vi "MISSION_ITEM Generic.vi"(11 "MISSION_ITEM":T1={"target_system"=0, "target_component"=0, "sequence"=0, "frame"=enum."GLOBAL RELATIVE ALT", "command"=0, "current"=FALSE, "autocontinue"=FALSE, "param1"=0.0, "param2"=0.0, "param3"=0.0, "param4"=0.0, "Lat"=0.0, "Lon"=0.0, "Altitude (m)"=0.0}) -> (3 "MAVLink Message":u8[](array[numeric]))   [LabVIEW 2014]
uses:
  Controls/Mission Planning Controls/MAVLINK Mission Item.ctl
  Controls/MAVLINK Mav Frame.ctl
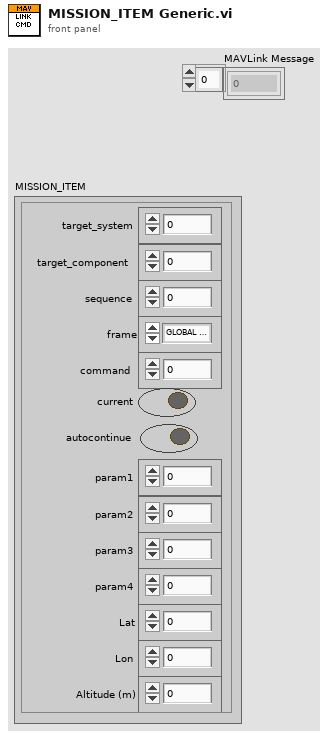
[diagram p1: front panel]
types:
  T1 = typedef "MAVLINK Mission Item.ctl" = cluster{"target_system":u8, "target_component":u8, "sequence":u16, "frame":T2, "command":u16, "current":bool, "autocontinue":bool, "param1":sgl, "param2":sgl, "param3":sgl, "param4":sgl, "Lat":sgl, "Lon":sgl, "Altitude (m)":sgl}
  T2 = typedef "MAVLINK Mav Frame.ctl" = enum8{"GLOBAL", "LOCAL NED", "MISSION", "GLOBAL RELATIVE ALT", "LOCAL ENU", "GLOBAL INT", "GLOBAL RELATIVE ALT INT", "LOCAL OFFSET NED", "BODY NED", "BODY OFFSET NED", "GLOBAL TERRAIN ALT", "GLOBAL TERRAIN ALT INT"}
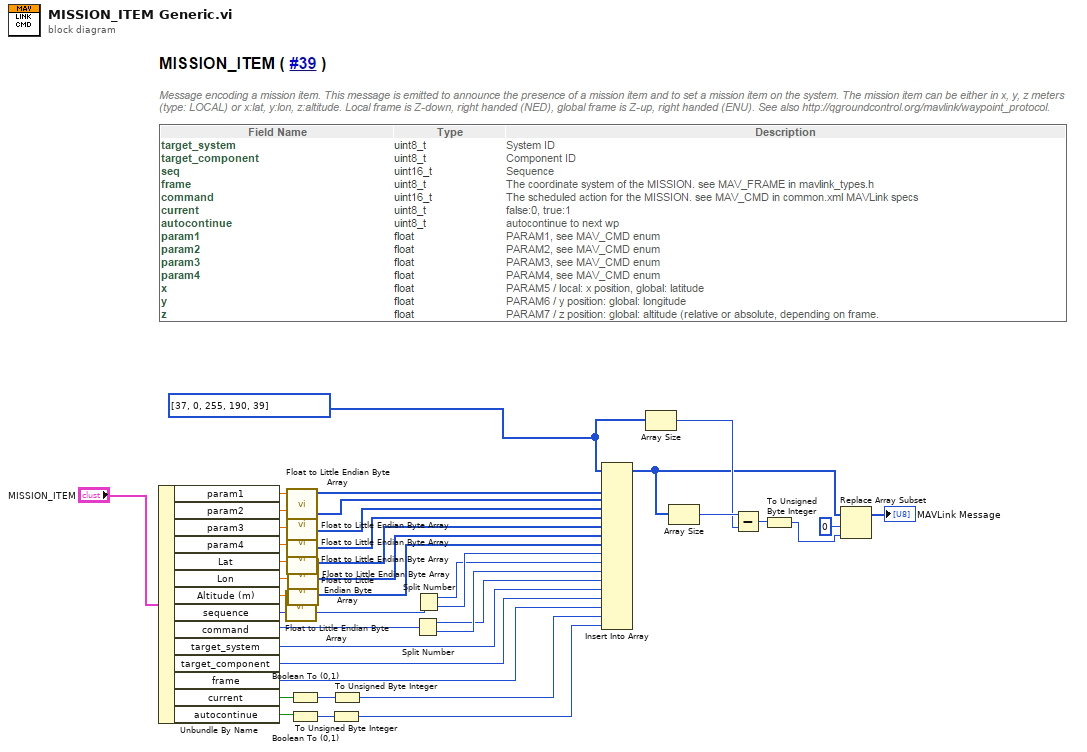
[diagram p0: block diagram]
diagram:
  w38 = u8[] [37, 0, 255, 190, 39]
  n1 = Unbundle By Name("MISSION_ITEM") -> ("param1"=w29:sgl, "param2"=w28:sgl, "param3"=w27:sgl, "param4"=w26:sgl, "Lat"=w25:sgl, "Lon"=w24:sgl, "Altitude (m)"=w23:sgl, "sequence"=w15:u16, "command"=w12:u16, "target_system"=w9:u8, "target_component"=w8:u8, "frame"=w7:T2, "current"=w6:bool, "autocontinue"=w5:bool)
  n2 = call "Float to Little Endian Byte Array.vi"("Float In"=w23) -> ("LE Byte Array"=w16:u8[])  [unwired: 10 in]
  n3 = call "Float to Little Endian Byte Array.vi"("Float In"=w29) -> ("LE Byte Array"=w22:u8[])  [unwired: 10 in]
  n4 = call "Float to Little Endian Byte Array.vi"("Float In"=w28) -> ("LE Byte Array"=w21:u8[])  [unwired: 10 in]
  n5 = call "Float to Little Endian Byte Array.vi"("Float In"=w27) -> ("LE Byte Array"=w20:u8[])  [unwired: 10 in]
  n6 = call "Float to Little Endian Byte Array.vi"("Float In"=w26) -> ("LE Byte Array"=w19:u8[])  [unwired: 10 in]
  n7 = call "Float to Little Endian Byte Array.vi"("Float In"=w25) -> ("LE Byte Array"=w18:u8[])  [unwired: 10 in]
  n8 = call "Float to Little Endian Byte Array.vi"("Float In"=w24) -> ("LE Byte Array"=w17:u8[])  [unwired: 10 in]
  n9 = Boolean To (0,1)(Boolean=w6) -> (0, 1=w4:i16)
  n10 = Boolean To (0,1)(Boolean=w5) -> (0, 1=w3:i16)
  n11 = To Unsigned Byte Integer(number=w3) -> (unsigned 8bit integer=w1:u8)
  n12 = To Unsigned Byte Integer(number=w4) -> (unsigned 8bit integer=w2:u8)
  n13 = Split Number(x=w12) -> (hi(x)=w10:u8, lo(x)=w11:u8)
  n14 = Split Number(x=w15) -> (hi(x)=w13:u8, lo(x)=w14:u8)
  n15 = Insert Into Array(array=w38, new element #1=w22, new element #2=w21, new element #3=w20, new element #4=w19, new element #5=w18, new element #6=w17, new element #7=w16, new element #8=w14, new element #9=w13, new element #10=w11, new element #11=w10, new element #12=w9, new element #13=w8, new element #14=w7, new element #15=w2, new element #16=w1) -> (w32:u8[])  [unwired: 1 in]
  n16 = Array Size(array=w38) -> (size(s)=w36:i32)
  n17 = Array Size(array=w32) -> (size(s)=w37:i32)
  n18 = Subtract(x=w37, y=w36) -> (x-y=w35:i32)
  n19 = To Unsigned Byte Integer(number=w35) -> (unsigned 8bit integer=w33:u8)
  n20 = Replace Array Subset(array=w32, new element=w33, index=0) -> (→"MAVLink Message":u8[])
